vi "MagX Get Probe Info.vi"(6 "Update experiment info file":bool, 7 "url":string="https://magfair.lanl.gov/rest/probs", 8 "error in":errorcluster, 11 "Station":string="Cell_3") -> (0 "error out":errorcluster, 3 "Data out":T1[](array[typedef]))   [LabVIEW 2024]
uses:
  Instrument info.ctl
  7bf855a0-2889-4335-a077-b20b33b30227.vi
  <vilib>/JDP Science/JSONtext/JSON text to Variant.vi
  <vilib>/JDP Science/JSONtext/LVClass Serializer/JSONtext LVClass Serializer.lvclass
  <vilib>/httpClient/LabVIEWHTTPClient.lvlib
panel:
  out "result string":string
  in  "Experiment info file":path=path "C:/Data/experiment_info.txt"
  out "body":string
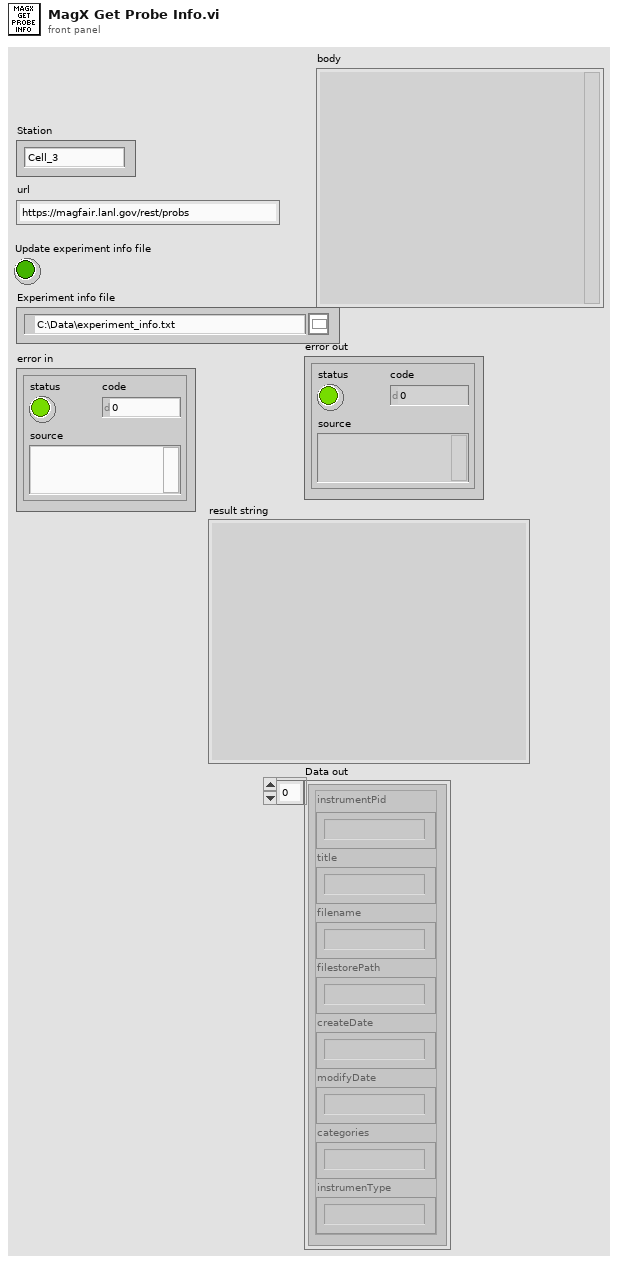
[diagram p1: front panel]
types:
  T1 = typedef "Instrument info.ctl" = cluster{"instrumentPid":string, "title":string, "filename":string, "filestorePath":string, "createDate":string, "modifyDate":string, "categories":string, "instrumenType":string}
  T2 = typedef "LabVIEWHTTPClient.lvlib/ClientHandle.ctl" = refnum<k1>
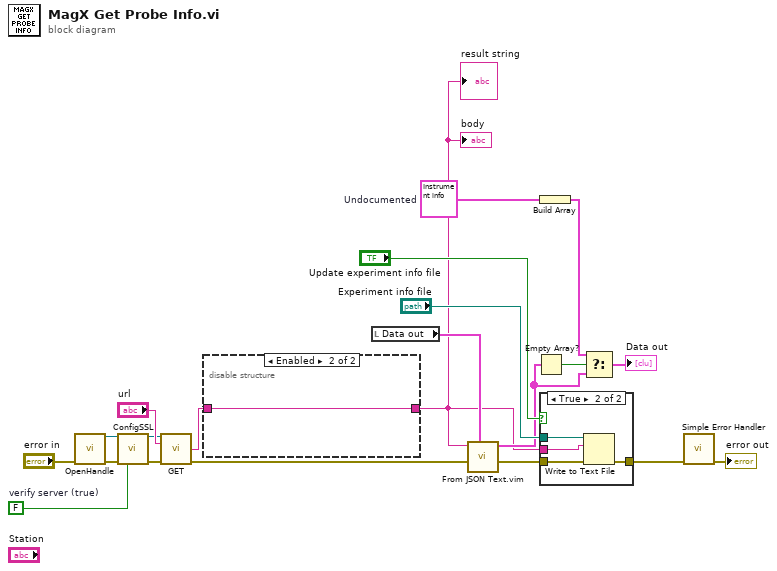
[diagram p0: block diagram]
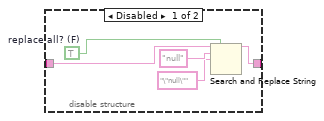
[diagram p2: hidden frame]
diagram:
  w8 = T1 {"instrumentPid"="Undocumented", "title"="Undocumented activity", "filename"="", "filestorePath"="", "createDate"="Undocumented activity", "modifyDate"="", "categories"="", "instrumenType"=""}  # Undocumented
  w9 = FALSE  # verify server (true)
  n1 = call <vilib>:"OpenHandle.vi"("error in (no error)"="error in") -> ("client handle out"=w13:T2, "error out"=w12:errorcluster)  [unwired: 13 in]
  n2 = call <vilib>:"ConfigSSL.vi"("client handle"=w13, "error in (no error)"=w12, "verify server (true)"=w9) -> ("client handle out"=w10:T2, "error out"=w11:errorcluster)  [unwired: 11 in]
  n3 = call <vilib>:"GET.vi"("client handle"=w10, "url"="url", "error in (no error)"=w11) -> ("body"=w2:string, "error out"=w20:errorcluster)  [unwired: 9 in, 2 out]
  n4 = disable-structure shown="Enabled" {
    disable-tunnel: w2 -> [w26 w27]
    disable-tunnel: [w23 w27] -> w1
    frame Disabled {
      w22 = TRUE  # replace all? (F)
      n5 = Search and Replace String(replace all?=w22, input string=w26, search string="null", replace string="\"null\"" ("search string")) -> (result string=w23:string)  [unwired: 4 in, 3 out]
    }
    frame Enabled {
    }
  }
  "body" <- w1
  "result string" <- w1
  n6 = local read "Data out"() -> (w4:T1[])
  n7 = call "From JSON Text.vim"("Data Type and Default Value"=w4, "error in (no error)"=w20, "JSON"=w1) -> ("error out"=w16:errorcluster, "Data out"=w3:T1[])  [unwired: 7 in]
  n8 = Empty Array?(array=w3) -> (empty?=w7:bool)
  n9 = Build Array(w8) -> (w6:T1[])
  n10 = case shown="True" "Update experiment info file" {
    tunnel: w16 -> [w28 w32]
    tunnel: "Experiment info file" -> [_ w31]
    tunnel: [w28 w30] -> w14
    tunnel: w1 -> [_ w29]
    frame False {
    }
    frame True {
      n11 = Write to Text File(file (use dialog)=w31, text=w29, error in=w32) -> (error out=w30:errorcluster)  [unwired: 1 in, 2 out]
    }
  }
  n12 = Select(t=w6, s=w7, f=w3) -> (s? t:f=→"Data out":T1[])
  n13 = call <vilib>:"Simple Error Handler.vi"("error in (no error)"=w14) -> ("error out"=→"error out":errorcluster)  [unwired: 4 in, 4 out]
